vi "table ignore input logic.vi"(7 "tag list":refnum<class "tag descriptor.lvclass">[](array[class]), 8 "CellPosition":T1, 10 "Table Control Reference":refnum<vi>, 11 "data type":refnum<vi>) -> (3 "Discard?":bool)   [LabVIEW 2013, in "PL Framework Configuration Tool.lvlib" / "EngineTags.lvclass"]
uses:
  EngineTags.lvclass
  <vilib>/NI/Tag Bus/tag/tag descriptor.lvclass
  <vilib>/Utility/miscctls.llb/LVRowAndColumnTypeDef.ctl
  <vilib>/NI/Tag Bus/tag/Data Type.ctl
  <vilib>/Utility/miscctls.llb/LVPositionTypeDef.ctl
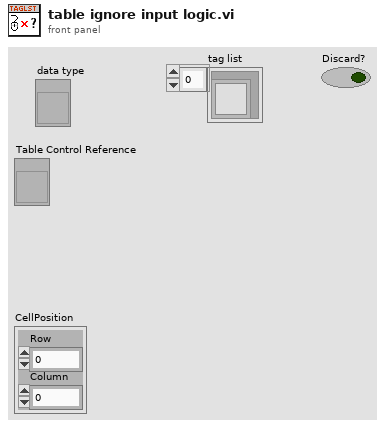
[diagram p1: front panel]
types:
  T1 = typedef "LVRowAndColumnTypeDef.ctl" = cluster{"Row":i32, "Column":i32}
  T2 = typedef "LVPositionTypeDef.ctl" = cluster{"Left":i32, "Top":i32}
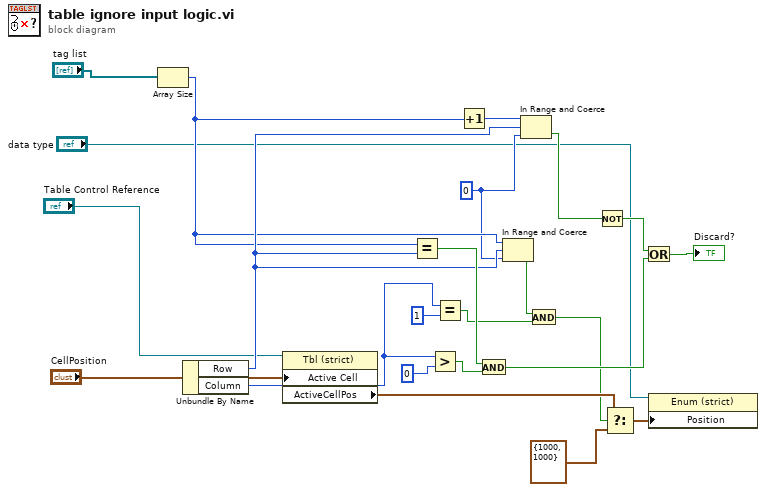
[diagram p0: block diagram]
diagram:
  w12 = 0 ("lower limit")
  n1 = Array Size(array="tag list") -> (size(s)=w15:i32)
  n2 = Unbundle By Name("CellPosition") -> ("Row"=w16:i32, "Column"=w18:i32)
  n3 = property class="Tbl (strict)"(reference="Table Control Reference", "Active Cell"="CellPosition") -> ("ActiveCellPos"=w9:T2)  [unwired: 1 in, 2 out]
  n4 = Equal?(x=w15, y=w16) -> (x = y?=w17:bool)
  n5 = Greater?(x=w18, y=0) -> (0:w20:bool)
  n6 = Equal?(x=w18, y=1) -> (x = y?=w6:bool)
  n7 = Increment(x=w15) -> (x+1=w13:i32)
  n8 = And(x=w17, y=w20) -> (x .and. y?=w22:bool)
  n9 = In Range and Coerce(upper limit=w15, x=w16, lower limit=w12) -> (In Range?=w11:bool)  [unwired: 1 out]
  n10 = In Range and Coerce(upper limit=w13, x=w16, lower limit=w12) -> (In Range?=w14:bool)  [unwired: 1 out]
  n11 = And(x=w11, y=w6) -> (x .and. y?=w7:bool)
  n12 = Not(x=w14) -> (.not. x?=w21:bool)
  n13 = Select(t=w9, s=w7, f=T2 {"Left"=1000, "Top"=1000} ("Position")) -> (s? t:f=w10:T2)
  n14 = Or(x=w21, y=w22) -> (x .or. y?=→"Discard?":bool)
  n15 = property on="Property Node" class="Enum (strict)"(reference="data type", "Position"=w10) -> ()  [unwired: 1 in, 2 out]
